vi "Run DDS clock.vi"() -> ()   [LabVIEW 2013]
uses:
  <instrlib>/niFgen/niFgen.llb/niFgen Waveform Type.ctl
panel:
  in  "stop":bool
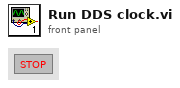
[diagram p1: front panel]
types:
  T1 = typedef "niFgen Waveform Type.ctl" = i32
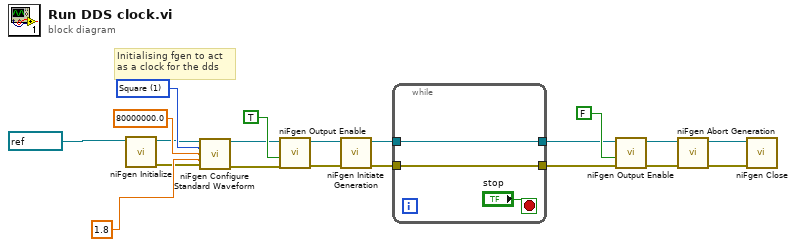
[diagram p0: block diagram]
diagram:
  w7 = T1 1 items=["Sine", "Square", "Triangle", "Ramp Up", "Ramp Down", "DC", "Noise", "User"] ("Waveform")
  # "Initialising fgen to act \nas a clock for the dds"
  n1 = call <instrlib>:"niFgen Initialize.vi"("Resource Name"=refnum<k15> "Dev1") -> ("error out"=w4:errorcluster, "Instrument Handle Out"=w3:refnum<k15>)  [unwired: 9 in]
  n2 = call <instrlib>:"niFgen Configure Standard Waveform.vi"("Instrument Handle"=w3, "Waveform"=w7, "Frequency"=80000000.0, "Amplitude"=1.8, "error in (no error)"=w4) -> ("Instrument Handle Out"=w2:refnum<k15>, "error out"=w1:errorcluster)  [unwired: 9 in]
  n3 = call <instrlib>:"niFgen Output Enable.vi"("error in (no error)"=w1, "Output Enable (default: True)"=TRUE, "Instrument Handle"=w2) -> ("error out"=w20:errorcluster, "Instrument Handle Out"=w19:refnum<k15>)  [unwired: 7 in]
  n4 = call <instrlib>:"niFgen Initiate Generation.vi"("error in (no error)"=w20, "Instrument Handle"=w19) -> ("error out"=w9:errorcluster, "Instrument Handle Out"=w11:refnum<k15>)  [unwired: 8 in]
  n5 = while {
    tunnel: [w22] -> w10
    tunnel: w11 -> [w22]
    tunnel: w9 -> [w21]
    tunnel: [w21] -> w8
    stop <- "stop" stop-if-true
  }
  n6 = call <instrlib>:"niFgen Output Enable.vi"("error in (no error)"=w8, "Output Enable (default: True)"=FALSE, "Instrument Handle"=w10) -> ("error out"=w17:errorcluster, "Instrument Handle Out"=w16:refnum<k15>)  [unwired: 7 in]
  n7 = call <instrlib>:"niFgen Abort Generation.vi"("error in (no error)"=w17, "Instrument Handle"=w16) -> ("error out"=w15:errorcluster, "Instrument Handle Out"=w14:refnum<k15>)  [unwired: 8 in]
  n8 = call <instrlib>:"niFgen Close.vi"("error in (no error)"=w15, "Instrument Handle"=w14) -> ()  [unwired: 9 in, 1 out]
